vi "PythonWrapper 2017.vi"(0 "file to run":path, 1 "expected output size (4096)":u32=4096, 2 "Python.exe":path=path "Python", 3 "data in":variant, 4 "run minimized? (T)":bool=TRUE) -> (5 "data out":variant, 6 "standard error":string, 7 "return code":i32, 8 "error out":errorcluster)   [LabVIEW 2017]
doc: "Allows for the passing of non-string data types to and from Python scripts."
uses:
  <vilib>/Utility/error.llb/DialogType.ctl
panel:
  in  "Show More":bool
  out "Flattened Output":string
  out "Flattened Input/bin file":string
  out "Raw Input":string
  out "Raw Output":string
  # "INPUTS"
  # "OUTPUTS"
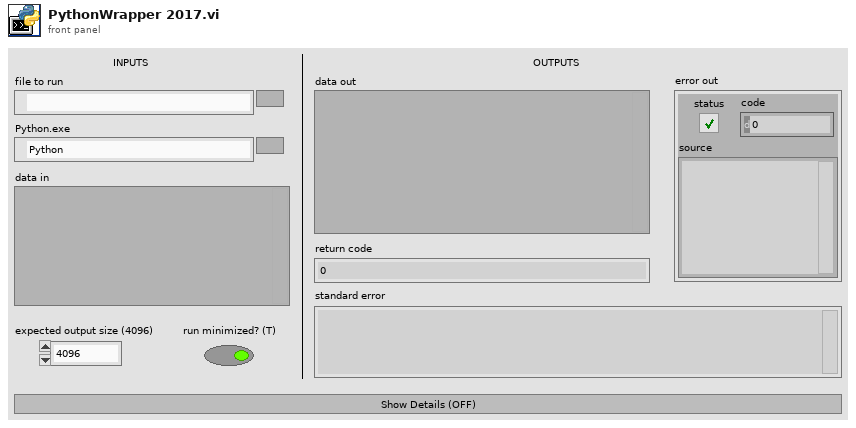
[diagram p1: front panel]
types:
  T1 = typedef "DialogType.ctl" = u16
  T2 = enum16{"big-endian, network order", "native, host order", "little-endian"}
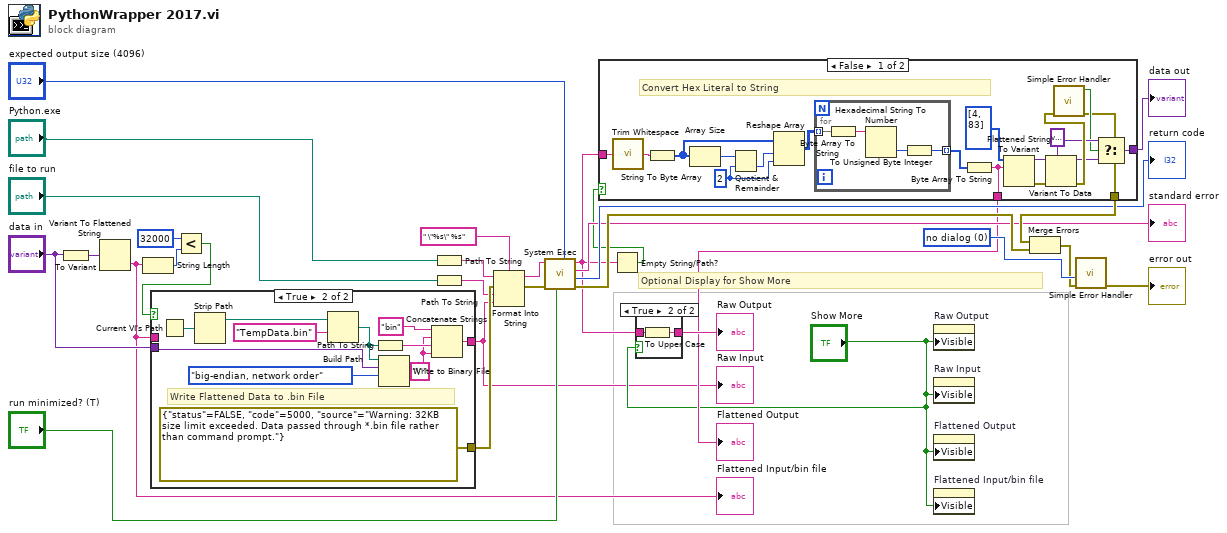
[diagram p0: block diagram]
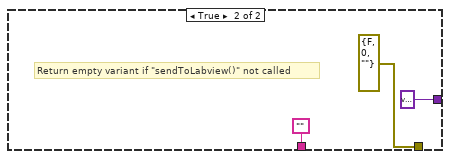
[diagram p2: hidden frame]
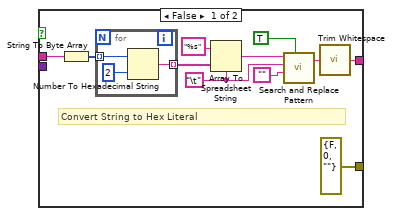
[diagram p3: hidden frame]
diagram:
  w15 = T1 0 items=["no dialog", "OK message", "continue or stop message", "OK message + warnings", "continue/stop + warnings"] ("type of dialog (OK msg:1)")
  # "Optional Display for Show More"
  n1 = To Variant(anything="data in") -> (Variant=w27:variant)
  n2 = Variant To Flattened String(Variant=w27) -> (data string=w12:string)  [unwired: 1 out]
  "Flattened Input/bin file" <- w12
  n3 = String Length(string=w12) -> (length=w10:i32)
  n4 = Less?(x=32000, y=w10) -> (x < y?=w9:bool)
  n5 = case shown="True" w9 {
    tunnel: "data in" -> [_ w51]
    tunnel: [w32 w48] -> w1
    tunnel: w12 -> [w33 _]
    tunnel: [errorcluster {"status"=FALSE, "code"=0, "source"=""} ("error constant") errorcluster {"status"=FALSE, "code"=5000, "source"="Warning: 32KB size limit exceeded. Data passed through *.bin file rather than command prompt."} ("error constant")] -> w30
    frame False {
      w38 = "\t"
      # "Convert String to Hex Literal"
      n6 = String To Byte Array(string=w33) -> (unsigned byte array=w41:u8[])
      n7 = for {
        tunnel: w41 -> [w43] mode=indexing
        tunnel: [w42] -> w34 mode=indexing
        n8 = Number To Hexadecimal String(1:2, 2:w43) -> (0:w42:string)
      }
      n9 = Array To Spreadsheet String(delimiter (Tab)=w38, array=w34, 3:"%s") -> (spreadsheet string=w39:string)
      n10 = call <vilib>:"Search and Replace Pattern.vi"("string"=w39, "regular expression (\"\")"=w38, "replace string (\"\")"="", "replace all? (F)"=TRUE) -> ("result string"=w35:string)  [unwired: 1 in, 1 out]
      n11 = call <vilib>:"Trim Whitespace.vi"("string"=w35) -> ("trimmed string"=w32:string)  [unwired: 1 in]
    }
    frame True {
      w47 = "\""
      # "Write Flattened Data to .bin File"
      n12 = Current VI's Path() -> (path=w54:path)
      n13 = Strip Path(path=w54) -> (stripped path=w55:path)  [unwired: 1 out]
      n14 = Build Path(base path=w55, name or relative path="TempData.bin") -> (appended path=w50:path)
      n15 = Path To String(path=w50) -> (string=w49:string)
      n16 = Write to Binary File(file (use dialog)=w50, data=w51, 9:T2."big-endian, network order" ("byte order (0:big-endian, network order)")) -> ()  [unwired: 3 in, 3 out]
      n17 = Concatenate Strings("bin", w47, w49, w47) -> (w48:string)
    }
  }
  "Raw Input" <- w1
  n18 = Path To String(path="Python.exe") -> (string=w26:string)
  n19 = Path To String(path="file to run") -> (string=w25:string)
  n20 = Format Into String(format string=" \"%s\" %s", initial string=w26, error in=w30, w25, w1) -> (resulting string=w2:string, error out=w23:errorcluster)
  n21 = call <vilib>:"System Exec.vi"("expected output size  (4096)"="expected output size (4096)", "run minimized? (F)"="run minimized? (T)", "error in (no error)"=w23, "command line"=w2) -> ("error out"=w28:errorcluster, "return code"=→"return code":i32, "standard error"=→"standard error":string, "standard output"=w8:string)  [unwired: 4 in]
  n22 = Empty String/Path?(string/path=w8) -> (empty?=w7:bool)
  n23 = case shown="False" w7 {
    tunnel: [w58 variant] -> w5
    tunnel: w8 -> [w63 _]
    tunnel: [w57 ""] -> w6
    tunnel: [w56 errorcluster {"status"=FALSE, "code"=0, "source"=""} ("error constant")] -> w29
    frame False {
      w71 = 2
      w60 = variant
      # "Convert Hex Literal to String"
      n24 = call <vilib>:"Trim Whitespace.vi"("string"=w63) -> ("trimmed string"=w65:string)  [unwired: 1 in]
      n25 = String To Byte Array(string=w65) -> (unsigned byte array=w69:u8[])
      n26 = Array Size(array=w69) -> (size(s)=w70:i32)
      n27 = Quotient & Remainder(x=w70, y=w71) -> (floor(x/y)=w72:i32)  [unwired: 1 out]
      n28 = Reshape Array(w69, w72, w71) -> (w68:u8[][])
      n29 = for {
        tunnel: w68 -> [w74] mode=indexing
        tunnel: [w75] -> w67 mode=indexing
        n30 = Byte Array To String(unsigned byte array=w74) -> (string=w77:string)
        n31 = Hexadecimal String To Number(string=w77) -> (number=w76:u32)  [unwired: 2 in, 1 out]
        n32 = To Unsigned Byte Integer(number=w76) -> (unsigned 8bit integer=w75:u8)
      }
      n33 = Byte Array To String(unsigned byte array=w67) -> (string=w57:string)
      n34 = Flattened String To Variant(6:w57, 7:i16[] [4, 83]) -> (0:w64:errorcluster, 3:w73:variant)  [unwired: 1 in]
      n35 = Variant To Data(error in=w64, type=w60, Variant=w73) -> (data=w61:variant, error out=w62:errorcluster)
      n36 = call <vilib>:"Simple Error Handler.vi"("error in (no error)"=w62) -> ("error?"=w59:bool, "error out"=w56:errorcluster)  [unwired: 4 in, 3 out]
      n37 = Select(t=w60, s=w59, f=w61) -> (s? t:f=w58:variant)
    }
    frame True {
      # "Return empty variant if \"sendToLabview()\" not called"
    }
  }
  "data out" <- w5
  "Flattened Output" <- w6
  n38 = case shown="True" "Show More" {
    tunnel: w8 -> [w81 w83]
    tunnel: [w81 w82] -> w16
    frame False {
    }
    frame True {
      n39 = To Upper Case(1:w83) -> (0:w82:string)
    }
  }
  "Raw Output" <- w16
  n40 = property on="Raw Output" class="Str"("Visible"="Show More") -> ()  [unwired: 2 in, 2 out]
  n41 = property on="Raw Input" class="Str"("Visible"="Show More") -> ()  [unwired: 2 in, 2 out]
  n42 = property on="Flattened Output" class="Str"("Visible"="Show More") -> ()  [unwired: 2 in, 2 out]
  n43 = property on="Flattened Input/bin file" class="Str"("Visible"="Show More") -> ()  [unwired: 2 in, 2 out]
  n44 = Merge Errors(w29, w28) -> (w4:errorcluster)
  n45 = call <vilib>:"Simple Error Handler.vi"("type of dialog (OK msg:1)"=w15, "error in (no error)"=w4) -> ("error out"=→"error out":errorcluster)  [unwired: 3 in, 4 out]
